vi "RequestTrig.vi"(8 "error in (no error)":errorcluster, 10 "Master Device in":refnum<class "Master Device.lvclass">, 11 "Aerotech_Soloist in":refnum<class "Aerotech_Soloist.lvclass">) -> (0 "error out":errorcluster, 2 "Master Device out":refnum<class "Master Device.lvclass">, 3 "Aerotech_Soloist out":refnum<class "Aerotech_Soloist.lvclass">)   [LabVIEW 2013, in "Aerotech_Soloist.lvclass"]
doc: "RequestTrig is the second subVI called in PrepareHWI--after ParseSWI.vi. Here, you should compare each ramp (end of last to start of first AND within each ramp) to see whether the device output is changing. For each ramp line, you should build a boolean array (reverse time order!) where TRUE denotes trigger required (i.e. output changes and must be triggered) and FALSE means no trigger is needed. Then pass the boolean array to Update Trigger Line.vi on the Master Device to request triggering.\n\nAfter all devices have a chance to request triggering, in FinalizeHWI.vi, each one will re-check their trigger line and Prune out lines which do not need to be programmed and then BuildHWI."
uses:
  Aerotech_Soloist.lvclass
  Master Device/Master Device.lvclass
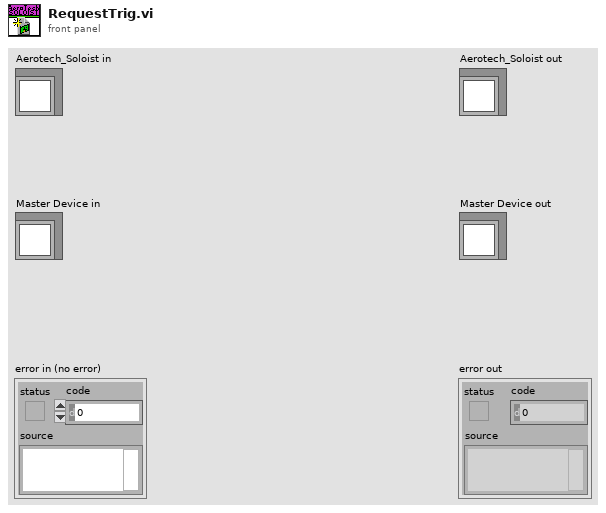
[diagram p1: front panel]
types:
  T1 = typedef "Aerotech_Soloist.lvclass/ParsedSWILine.ctl" = cluster{"ParameterScript":string, "CommandScript":string}
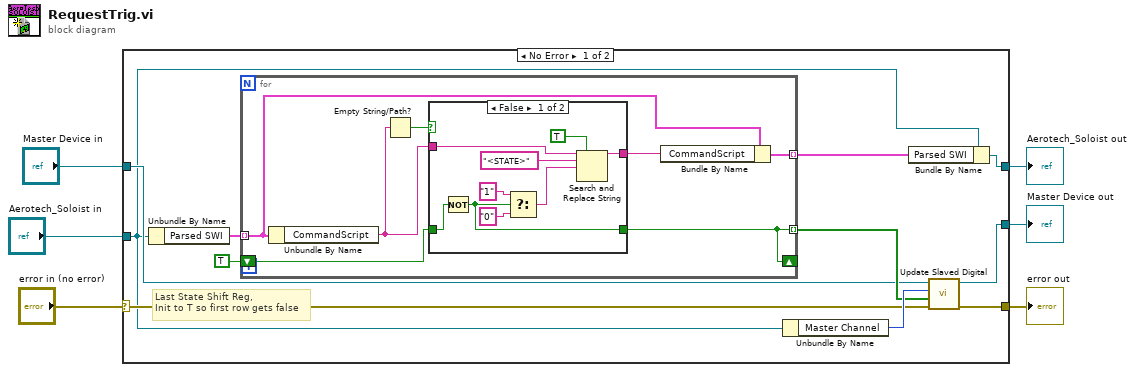
[diagram p0: block diagram]
diagram:
  n1 = case shown="No Error" "error in (no error)" {
    selector: "error in (no error)" -> [w10 w38]
    tunnel: [w17 w36] -> w1
    tunnel: [w12 w38] -> w6
    tunnel: "Aerotech_Soloist in" -> [w9 w37]
    tunnel: "Master Device in" -> [w11 w36]
    tunnel: [w8 w37] -> w2
    frame No Error {
      # "Last State Shift Reg,\nInit to T so first row gets false"
      n2 = Unbundle By Name(w9) -> ("Parsed SWI"=w15:T1[])
      n3 = for {
        tunnel: w15 -> [w20] mode=indexing
        shift-right: [w22] -> _
        shift-left: TRUE -> [w23]
        tunnel: [w22] -> w13 mode=indexing
        tunnel: [w18] -> w7 mode=indexing
        n4 = Unbundle By Name(w20) -> ("CommandScript"=w21:string)
        n5 = Empty String/Path?(string/path=w21) -> (empty?=w24:bool)
        n6 = case shown="False" w24 {
          tunnel: w23 -> [w33 w35]
          tunnel: [w28 w35] -> w22
          tunnel: w21 -> [w32 w34]
          tunnel: [w30 w34] -> w19
          frame False {
            n7 = Not(x=w33) -> (.not. x?=w28:bool)
            n8 = Select(t="1" ("search string"), s=w28, f="0" ("search string")) -> (s? t:f=w25:string)
            n9 = Search and Replace String(replace all?=TRUE ("replace all? (F)"), input string=w32, search string="<STATE>", replace string=w25) -> (result string=w30:string)  [unwired: 4 in, 3 out]
          }
          frame True {
          }
        }
        n10 = Bundle By Name(cluster=w20, "CommandScript"=w19) -> (w18:T1)
      }
      n11 = Unbundle By Name(w9) -> ("Master Channel"=w16:i32)
      n12 = Bundle By Name(cluster=w9, "Parsed SWI"=w7) -> (w8:refnum<class "Aerotech_Soloist.lvclass">)
      n13 = call-dynamic "Update Slaved Digital.vi"("error in (no error)"=w10, "Output States"=w13, "Master Channel Number"=w16, "Master Device in"=w11) -> ("error out"=w12:errorcluster, "Master Device out"=w17:refnum<class "Master Device.lvclass">)  [unwired: 6 in]
    }
    frame Error {
    }
  }
  "error out" <- w6
  "Aerotech_Soloist out" <- w2
  "Master Device out" <- w1
